vi "NI VeriStand - Commit System Explorer Update Buffer Wrapper.vi"(8 "error in":errorcluster) -> (0 "error out":errorcluster)   [LabVIEW 2019, in "DSF System Explorer.lvlib"]
uses:
  DSF System Explorer.lvlib
  <vilib>/NI VeriStand/Custom Device API/Custom Device API.lvlib
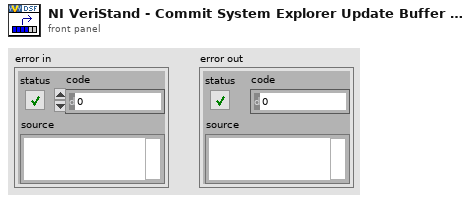
[diagram p1: front panel]
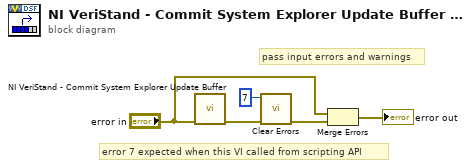
[diagram p0: block diagram]
diagram:
  # "error 7 expected when this VI called from scripting API"
  # "pass input errors and warnings"
  n1 = call <vilib>:"NI VeriStand - Commit System Explorer Update Buffer.vi"("error in (no error)"="error in") -> ("error out"=w4:errorcluster)  [unwired: 10 in]
  n2 = call <vilib>:"Clear Errors.vi"("error in (no error)"=w4, "specific error code to clear (0: all)"=7) -> ("error out"=w2:errorcluster)  [unwired: 4 in, 1 out]
  n3 = Merge Errors("error in", w2) -> (→"error out":errorcluster)
